vi "DMA.Scatter-Gather.Initialize.vi"   [LabVIEW 2016, in "GE 5565PIORC.lvclass"]
uses:
  GE 5565PIORC.lvclass
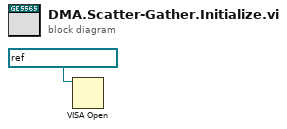
[diagram p0: block diagram]
diagram:
  n1 = VISA Open(VISA resource name=refnum<visa-resource-name> "PXI0::MEMACC") -> ()  [unwired: 4 in, 2 out]
